vi "LS218-TempTester.vi"(11 "error in (no error)":errorcluster) -> ()   [LabVIEW 2012]
doc: "This VI was designed to demonstrate typical usage of sub VIs containing the more common 218 functions. The VI Initializes the instrument, calls the Application Temperature Monitor VI, and then closes the instrument. The Application Temperature Monitor VI first configures the input group and input to be read using the LSCI 218 Config input.vi. Time is then provided for the instrument to configure the input group and input. Finally, the selected input is read."
uses:
  <instrlib>/Lake Shore Cryotronics 218/Lake Shore Cryotronics 218.lvlib
panel:
  in  "SelectComPort":refnum<visa-resource-name>
  out "readings":dbl[](array[numeric])=[32.523, 38.795, 23.185, 32.195, -245.15, -245.15, -245.15, -245.15]
  in  "stop":bool=TRUE
  out "error out":errorcluster={"status"=FALSE, "code"=1073676418, "source"="VISA Close in MON_LS218_Init.vi->LS218-TempTester.vi"}
  out "VISA Out":refnum<visa-resource-name>="ASRL5::INSTR"
  out "*IDN?":string="LSCI,MODEL218S,219303,020602\r"
  # "Firt Select \"SelectComPort\" , then Click Run.  To stop GUI,  click \" Press to EXIT\""
  # "LakeShore 218 Temperature Tester"
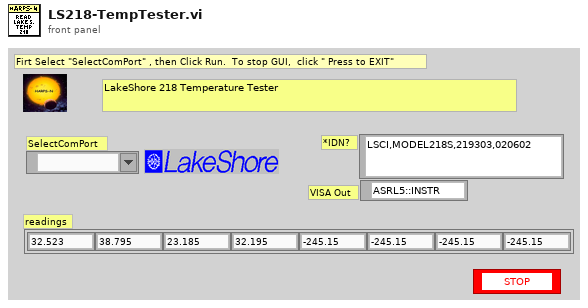
[diagram p1: front panel]
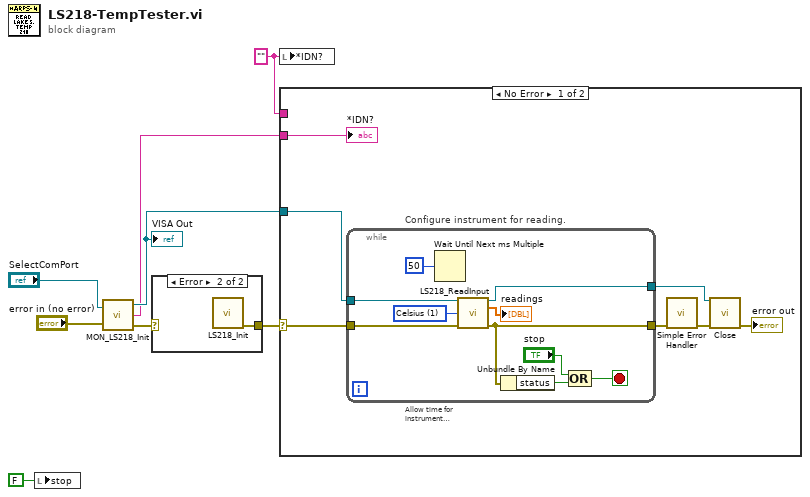
[diagram p0: block diagram]
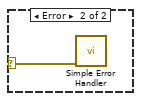
[diagram p3: hidden frame]
diagram:
  w6 = "" ("reply")
  n1 = local write "stop"(FALSE ("stop")) -> ()
  n2 = call "MON_LS218_Init.vi"("error in (no error)"="error in (no error)", "found VISA"="SelectComPort") -> ("error out"=w3:errorcluster, "Reply"=w1:string, "VISA Out"=w2:refnum<visa-resource-name>)
  "VISA Out" <- w2
  n3 = case shown="Error" w3 {
    selector: w3 -> [w9 _]
    tunnel: [w9 w10] -> w5
    frame No Error {
    }
    frame Error {
      n4 = call <instrlib>:"LS218_Init.vi"() -> ("error out"=w10:errorcluster)  [unwired: 13 in, 2 out]
    }
  }
  n5 = local write "*IDN?"(w6) -> ()
  n6 = case shown="No Error" w5 {
    selector: w5 -> [w11 w28]
    tunnel: w2 -> [w17 _]
    tunnel: w1 -> [w12 _]
    tunnel: w6 -> [_ _]
    frame No Error {
      # "Allow time for instrument \nto initialize."
      # "Configure instrument for reading."
      n7 = while {
        tunnel: w17 -> [w24]
        tunnel: [w26] -> w16
        tunnel: [w23] -> w15
        tunnel: w11 -> [w22]
        stop <- w18 stop-if-true
        w25 = u16 1 items=["Kelvin", "Celsius", "Sensor Units", "Linear Data"] ("Data Source")
        n8 = Wait Until Next ms Multiple(millisecond multiple=u32 50) -> ()  [unwired: 1 out]
        n9 = call <instrlib>:"LS218_ReadInput.vi"("VISA"=w24, "Data Source"=w25, "error in"=w22) -> ("VISA out"=w23:refnum<visa-resource-name>, "InputArray"=→"readings":dbl[], "error out"=w26:errorcluster)  [unwired: 10 in]
        n10 = Unbundle By Name(w26) -> ("status"=w19:bool)
        n11 = Compound Arithmetic op=OR("stop", w19) -> (w18:bool)
      }
      n12 = call <vilib>:"Simple Error Handler.vi"("error in (no error)"=w16) -> ("error out"=w14:errorcluster)  [unwired: 4 in, 4 out]
      n13 = call <instrlib>:"Close.vi"("VISA resource name"=w15, "error in (no error)"=w14) -> ("error out"=→"error out":errorcluster)  [unwired: 13 in]
      "*IDN?" <- w12
    }
    frame Error {
      n14 = call <vilib>:"Simple Error Handler.vi"("error in (no error)"=w28) -> ()  [unwired: 4 in, 5 out]
    }
  }
